vi "HMI_Menu.vi"(11 "Menu Items":T1) -> ()   [LabVIEW 2024]
uses:
  Control Definitions/Def_MenuItems.ctl
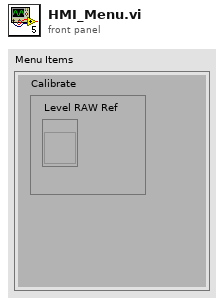
[diagram p1: front panel]
types:
  T1 = typedef "Def_MenuItems.ctl" = cluster{"Calibrate":cluster{"Level RAW Ref":refnum<vi>}}
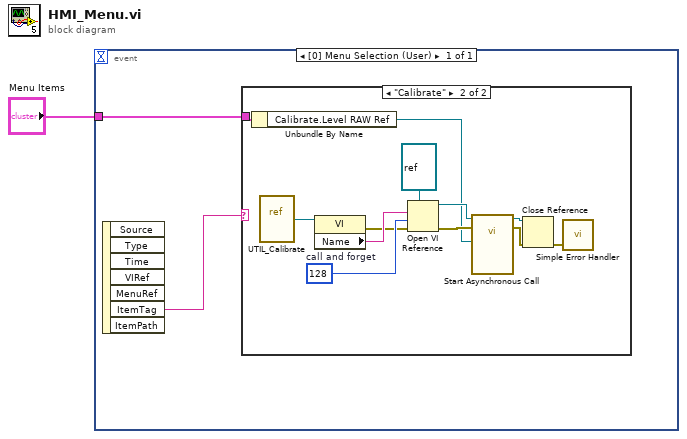
[diagram p0: block diagram]
diagram:
  n1 = event shown="[0] Menu Selection (User)" {
    selector: _ -> [_]
    dyn-events: _ -> [_]
    timeout: _ -> [_]
    tunnel: "Menu Items" -> [w2]
    event Menu Selection (User) {
      n2 = event-data() -> ("ItemTag"=w3:string)  [unwired: 1 in, 6 out]
      n3 = case shown="\"Calibrate\"" w3 {
        tunnel: w2 -> [_ w5]
        frame "False", Default {
        }
        frame "Calibrate" {
          w15 = 128  # call and forget
          n4 = Unbundle By Name(w5) -> ("Calibrate.Level RAW Ref"=w4:refnum<vi>)
          n5 = vi-ref "UTIL_Calibrate.vi"() -> (w8:refnum<vi>)
          n6 = property class="VI"(reference=w8) -> (error out=w6:errorcluster, "Name"=w7:string)  [unwired: 1 in, 1 out]
          n7 = Open VI Reference(type specifier VI Refnum (for type only)=refnum<vi> refnum, vi path=w7, options=w15, error in (no error)=w6) -> (vi reference=w13:refnum<vi>, error out=w12:errorcluster)  [unwired: 2 in]
          n8 = call-by-ref "Start Asynchronous Call"(reference=w13, error in=w12, "Digital in"=w4) -> (reference out=w10:refnum<vi>, error out=w11:errorcluster)  [unwired: 10 in, 1 out]
          n9 = Close Reference(reference=w10, error in (no error)=w11) -> (error out=w9:errorcluster)
          n10 = call <vilib>:"Simple Error Handler.vi"("error in (no error)"=w9) -> ()  [unwired: 4 in, 5 out]
        }
      }
    }
  }
